vi "Read JSON Config.vi"(8 "error in (no error)":errorcluster, 10 "JSON Config":string, 11 "Concatenate_STR in":refnum<class "Concatenate_STR.lvclass">) -> (0 "error out":errorcluster, 3 "Concatenate_STR out":refnum<class "Concatenate_STR.lvclass">)   [LabVIEW 2021, in "Concatenate_STR.lvclass"]
uses:
  Concatenate_STR.lvclass
  C:/Program Files (x86)/National Instruments/LabVIEW 2021/vi.lib/TSA/Abstract Data Classes/Abs_Types/Type/Abs_Type.lvclass
  Concatenate_STR.lvclass/Concatenate_STR.ctl
  Abs_Types/String/Abs_String.lvclass
  C:/Program Files (x86)/National Instruments/LabVIEW 2021/vi.lib/TSA/Abstract Data Classes/Abs_Types/Value/Abs_Value.lvclass
  <vilib>/Utility/LVClass/Get LV Class Name.vi
  Abs_Types/Type/Abs_Type.lvclass
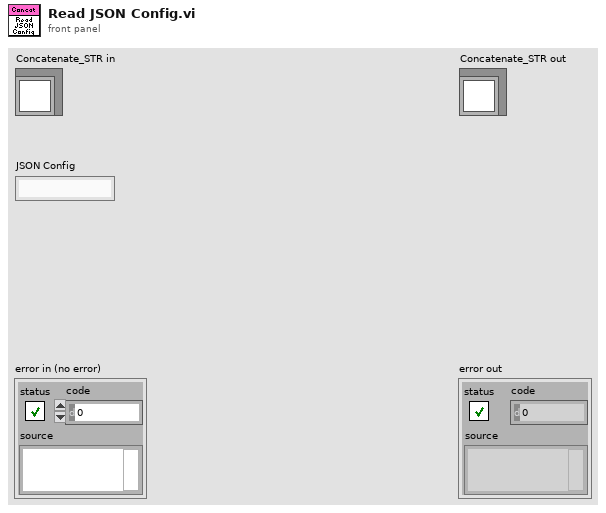
[diagram p1: front panel]
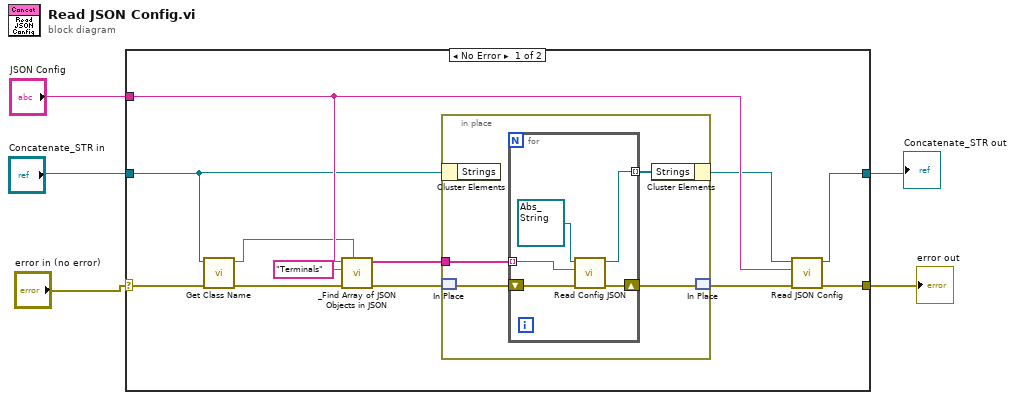
[diagram p0: block diagram]
diagram:
  n1 = case shown="No Error" "error in (no error)" {
    selector: "error in (no error)" -> [w13 w27]
    tunnel: [w17 w27] -> w1
    tunnel: [w16 w28] -> w2
    tunnel: "JSON Config" -> [w15 _]
    tunnel: "Concatenate_STR in" -> [w12 w28]
    frame No Error {
      n2 = call "Get Class Name.vi"("error in (no error)"=w13, "Abs_Type in"=w12) -> ("error out"=w14:errorcluster, "class name"=w7:string)  [unwired: 8 in]
      n3 = call "_Find Array of JSON Objects in JSON.vi"("JSON Object Name"=w7, "error in (no error)"=w14, "JSON Array Name"="Terminals", "JSON Config"=w15) -> ("error out"=w11:errorcluster, "JSON Objects"=w10:string[])  [unwired: 6 in]
      n4 = in-place {
        in-place-border: w10 -> [w21]
        n5 = in-place-cluster #1(w12) -> ()  [unwired: 1 out]
        n6 = in-place-match #2(w11) -> (w20:errorcluster)
        n7 = for {
          tunnel: w21 -> [w26] mode=indexing
          tunnel: [w23] -> w18 mode=indexing
          shift-right: [w24] -> w19
          shift-left: w20 -> [w25]
          n8 = call "Read Config JSON.vi"("error in (no error)"=w25, "JSON Config"=w26, "Abs_Type in"=refnum<class "Abs_String.lvclass"> refnum ("String")) -> ("error out"=w24:errorcluster, "Abs_Type out"=w23:refnum<class "Abs_String.lvclass">)  [unwired: 7 in]
        }
        n9 = in-place-cluster #1("Strings"=w18) -> (w8:refnum<class "Concatenate_STR.lvclass">)
        n10 = in-place-match #2(w19) -> (w9:errorcluster)
      }
      n11 = call-parent "Read JSON Config.vi"("error in (no error)"=w9, "JSON Config"=w15, "Abs_Type in"=w8) -> ("error out"=w17:errorcluster, "Abs_Type out"=w16:refnum<class "Concatenate_STR.lvclass">)  [unwired: 7 in]
    }
    frame Error {
    }
  }
  "error out" <- w1
  "Concatenate_STR out" <- w2
